vi "O2 RT Test.vi"() -> ()   [LabVIEW 2011]
uses:
  <vilib>/Platform/TimedLoop/XDataNode/timing_clust.ctl
  <vilib>/Platform/TimedLoop/XDataNode/nitl_modes.ctl
  <vilib>/Platform/TimedLoop/XDataNode/wakeup.ctl
  <vilib>/FPGAPlugInAG/cRIO-9074/niLvFpga_Open_cRIO-9074.vi
  <vilib>/rvi/interface/common/dynamic/niFpgaDynamicAddResources.vi
  <vilib>/Utility/error.llb/Error Cluster From Error Code.vi
  <vilib>/rvi/errors/niLvFpgaAdjustHostInterfaceError.vi
  <vilib>/FPGAPlugInAG/Dynamic/niLvFpga_Close_Dynamic.vi
  <vilib>/Platform/TimedLoop/XDataNode/XDataNode.xnode
  <vilib>/rvi/interface/nirviOpenFPGA/nirviOpenFPGA.xnode
  FPGA Bitfiles/MAXCAT_FPGATarget2_O2test_344E535A.lvbitx
  O2 test.vi
  <vilib>/rvi/interface/nirviReadWriteControl/nirviReadWriteControl.xnode
  <vilib>/rvi/interface/nirviCloseFPGA/nirviCloseFPGA.xnode
  <vilib>/Platform/TimedLoop/XDataNode/XDNodeRunTimeDep.lvlib
  NiFpgaLv.dll
  <vilib>/rvi/interface/Simulation/niFpgaSimulationCallBeginRW.vi
panel:
  out "FPGA Error Out":errorcluster
  in  "Stop":bool
  out "Lambda Chart":T1(graph)
  in  "UEGOModuleEnable":bool
  in  "UEGO Back Pressure (bar)":T2={"UEGO1BackPressure (bar)"=1.013, "UEGO2BackPressure (bar)"=1.013}
  in  "SensorEnable":T3
  out "UEGO Sensor Results":T4={"UEGO1Lambda"=1.0036743, "UEGO1Phi"=1.0, "UEGO1AFRatio"=14.7, "UEGO1Ip (mA)"=0.0, "UEGO2Lambda"=1.0033587, "UEGO2Phi"=1.0, "UEGO2AFRatio"=14.7, "UEGO2Ip (mA)"=0.0} {"UEGO1Lambda" scale=0.7..1.3; "UEGO2Lambda" scale=0.7..1.3}
  out "EGO Sensor Results":T5 {"EGO4Status" items=["COLD SENSOR", "FOULED SENSOR", "RICH", "LEAN"]; "EGO3Status" items=["COLD SENSOR", "FOULED SENSOR", "RICH", "LEAN"]; "EGO2Status" items=["COLD SENSOR", "FOULED SENSOR", "RICH", "LEAN"]; "EGO1Status" items=["COLD SENSOR", "FOULED SENSOR", "RICH", "LEAN"]}
  out "UEGO Temperature (C)":T6
  out "UEGO Heater Duty Cycle (%)":T7
  out "UEGO Diagnostics":T8={"ModulePresent"=FALSE, "UEGO1SensorFault"=63, "UEGO2SensorFault"=63, "UEGO1HeaterFault"=192, "UEGO2HeaterFault"=192, "UEGOFuseStatus"=0, "Battery (V)"=0.0} {"UEGOFuseStatus" items=["FUSE OK", "FUSE BLOWN"]; "UEGO2SensorFault" items=["NO FAULT"=63, "SHORT TO GND OR BATT"=0]; "UEGO2HeaterFault" items=["SHORT TO GROUND"=0, "OPEN CIRCUIT"=64, "SHORT TO BATTERY"=128, "NO FAULT"=192]; "UEGO1SensorFault" items=["NO FAULT"=63, "SHORT TO GND OR BATT"=0]; "UEGO1HeaterFault" items=["SHORT TO GROUND"=0, "OPEN CIRCUIT"=64, "SHORT TO BATTERY"=128, "NO FAULT"=192]}
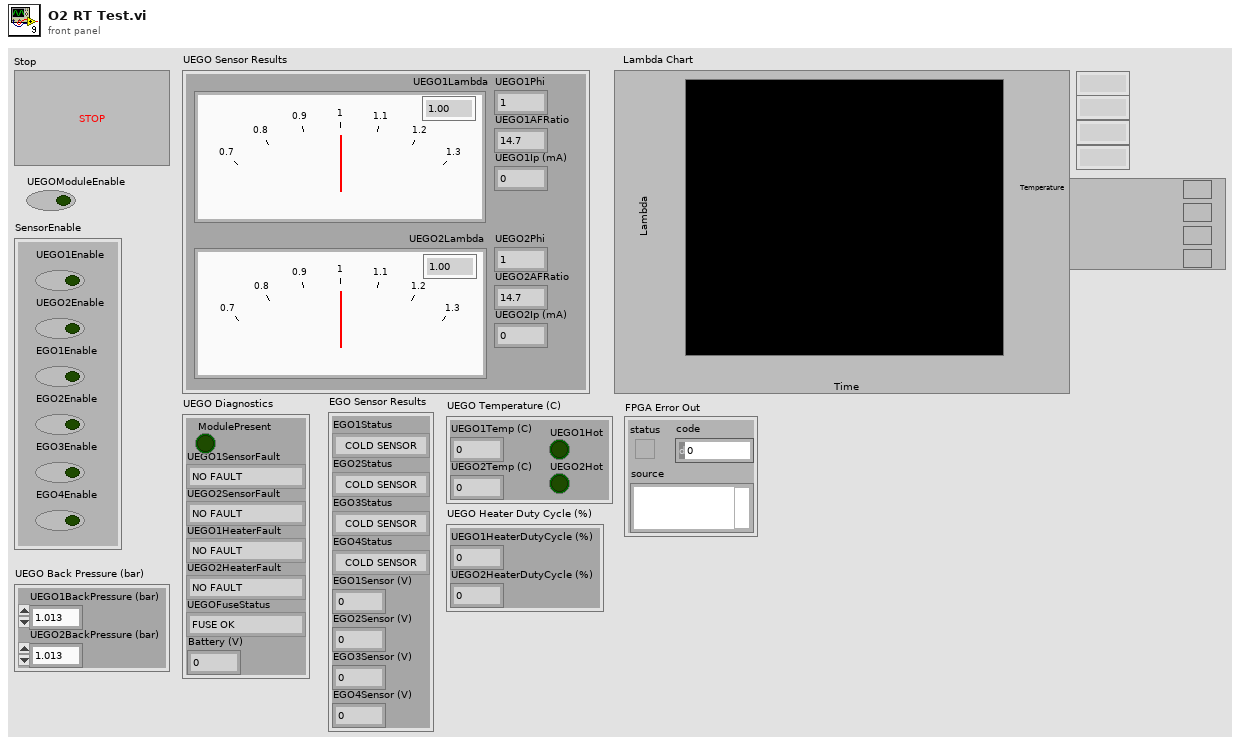
[diagram p1: front panel]
types:
  T1 = cluster{"UEGO1Lambda":sgl, "UEGO2Lambda":sgl, "UEGO1Temp (C)":sgl, "UEGO2Temp (C)":sgl}
  T2 = cluster{"UEGO1BackPressure (bar)":sgl, "UEGO2BackPressure (bar)":sgl}
  T3 = cluster{"UEGO1Enable":bool, "UEGO2Enable":bool, "EGO1Enable":bool, "EGO2Enable":bool, "EGO3Enable":bool, "EGO4Enable":bool}
  T4 = cluster{"UEGO1Lambda":sgl, "UEGO1Phi":sgl, "UEGO1AFRatio":sgl, "UEGO1Ip (mA)":sgl, "UEGO2Lambda":sgl, "UEGO2Phi":sgl, "UEGO2AFRatio":sgl, "UEGO2Ip (mA)":sgl}
  T5 = cluster{"EGO1Status":u8, "EGO2Status":u8, "EGO3Status":u8, "EGO4Status":u8, "EGO1Sensor (V)":sgl, "EGO2Sensor (V)":sgl, "EGO3Sensor (V)":sgl, "EGO4Sensor (V)":sgl}
  T6 = cluster{"UEGO1Temp (C)":sgl, "UEGO2Temp (C)":sgl, "UEGO1Hot":bool, "UEGO2Hot":bool}
  T7 = cluster{"UEGO1HeaterDutyCycle (%)":sgl, "UEGO2HeaterDutyCycle (%)":sgl}
  T8 = cluster{"ModulePresent":bool, "UEGO1SensorFault":u8, "UEGO2SensorFault":u8, "UEGO1HeaterFault":u8, "UEGO2HeaterFault":u8, "UEGOFuseStatus":u8, "Battery (V)":sgl}
  T9 = typedef "XDNodeRunTimeDep.lvlib/timing_clust.ctl" = cluster{"Expected End [f-1]":u64, "Actual End [f-1]":u64, "Finished Late? [f-1]":bool, "Expected End [i-1]":u64, "Actual End [i-1]":u64, "Finished Late? [i-1]":bool, "Expected Start [i]":u64, "Actual Start [i]":u64, "Expected Start [f]":u64, "Actual Start [f]":u64, "Source Name":string, "Structure Name":string, "Period":i64, "Deadline":i64, "Offset":i64, "Start":i64, "Priority":i32, "Timeout":i32, "Mode":T10, "Wakeup Reason":T11, "Error":errorcluster, "Source Type":string, "Secondary Source Type":string, "Global End Time":u64, "Global Start Time":u64, "Frame Duration":u64, "Iteration Duration":u64, "Assigned CPU":i32, "I/O Scan Engine Mode":u32}
  T10 = typedef "XDNodeRunTimeDep.lvlib/nitl_modes.ctl" = enum32{"No Change", "Process missed periods, maintain original phase", "Discard missed periods, maintain original phase", "Process missed periods, ignore original phase", "Discard missed periods, ignore original phase"}
  T11 = typedef "XDNodeRunTimeDep.lvlib/wakeup.ctl" = enum32{"Normal", "Aborted", "Asynchronous wakeup", "Timing source error", "Timed loop error", "Timeout"}
  T12 = cluster{"Stoich A/F Ratio":sgl, "IpArray (mA)":sgl[], "LambdaArray":sgl[]}
  T13 = cluster{"UEGO1Diag":u8, "UEGO2Diag":u8, "UEGO1Sensor":i16, "UEGO2Sensor":i16, "UEGO1Heater":i16, "UEGO2Heater":i16, "UEGO1AmpOffset":i16, "UEGO2AmpOffset":i16, "UEGO1RIOffset":i16, "UEGO2RIOffset":i16, "UEGO1HeaterGain":i16, "UEGO2HeaterGain":i16, "Fuse":i16, "EGO1Sensor":i16, "EGO2Sensor":i16, "EGO3Sensor":i16, "EGO4Sensor":i16, "Battery":i16, "ModulePresent":bool, "UEGO1ID":u8, "UEGO2ID":u8}
  T14 = cluster{"ModuleEnable":bool, "WatchdogIn":bool, "UEGO1Hot":bool, "UEGO2Hot":bool, "Cal1Request":bool, "Cal2Request":bool, "UEGOHeaterPeriod":u16, "UEGO1HeaterPulseWidth":u16, "UEGO2HeaterPulseWidth":u16}
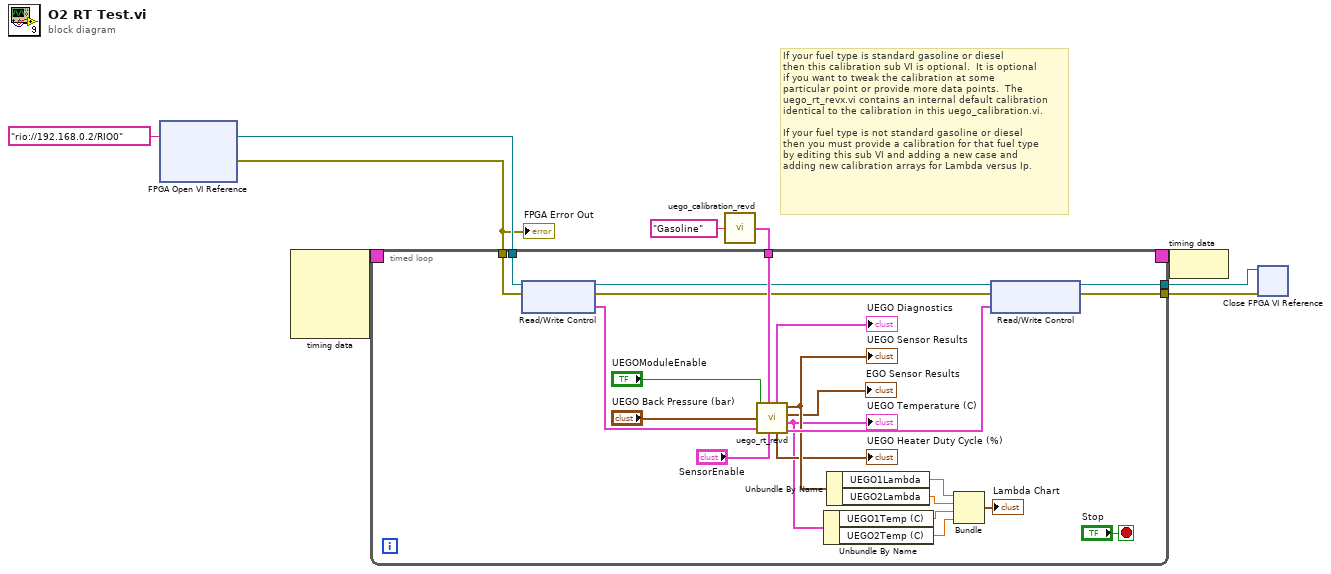
[diagram p0: block diagram]
diagram:
  # "If your fuel type is standard gasoline or diesel\nthen this calibration sub VI is optional.  It is optional \nif you want to tweak the calibration at some \nparticular point or provide more data points.  The \nuego_rt_revx.vi contains an internal default calibration\nidentical to the calibration in this uego_calibration.vi.\n\nIf your fuel type is not standard gasoline or diesel\nthen you must provide a calibration for that fuel type\nby editing this sub VI and adding a new case and \nadding new calibration arrays for Lambda versus Ip."
  n1 = xnode "FPGA Open VI Reference"("resource name"=tag "rio://192.168.0.2/RIO0") -> ("FPGA VI Reference Out"=w6:refnum<k20>, "error out"=w5:errorcluster)  [unwired: 1 in]
  "FPGA Error Out" <- w5
  n2 = node-c288() -> (w9:T9)  [unwired: 4 out]
  n3 = call <vilib>:"uego_calibration_revd.vi"("Fuel Selection"="Gasoline") -> ("UEGOCalibration"=w7:T12)
  n4 = timed-loop {
    tunnel: w5 -> [w29]
    tunnel: w7 -> [w31]
    tunnel: w6 -> [w32]
    timing-out: [_] -> w8
    timing: w9 -> [_]
    tunnel: [w20] -> w4
    tunnel: [w19] -> w3
    stop <- "Stop" stop-if-true
    n5 = xnode "Read/Write Control"("FPGA VI Reference In"=w32, "error in"=w29) -> ("FPGA VI Reference Out"=w30:refnum<k20>, "error out"=w28:errorcluster, "UEGOData"=w22:T13)
    n6 = call <vilib>:"uego_rt_revd.vi"("UEGOModuleEnable"="UEGOModuleEnable", "UEGOCalibration"=w31, "UEGO Back Pressure (bar)"="UEGO Back Pressure (bar)", "UEGOData (From FPGA)"=w22, "SensorEnable"="SensorEnable") -> ("UEGO Diagnostics"=→"UEGO Diagnostics":T8, "UEGO Sensor Results"=w21:T4, "EGO Sensor Results"=→"EGO Sensor Results":T5, "UEGO Heater Duty Cycle (%)"=→"UEGO Heater Duty Cycle (%)":T7, "UEGO Temperature (C)"=w13:T6, "UEGOControl (To FPGA)"=w23:T14)
    "UEGO Sensor Results" <- w21
    "UEGO Temperature (C)" <- w13
    n7 = Unbundle By Name(w13) -> ("UEGO1Temp (C)"=w12:sgl, "UEGO2Temp (C)"=w11:sgl)
    n8 = Unbundle By Name(w21) -> ("UEGO1Lambda"=w25:sgl, "UEGO2Lambda"=w24:sgl)
    n9 = Bundle("UEGO1Lambda"=w25, "UEGO2Lambda"=w24, "UEGO1Temp (C)"=w12, "UEGO2Temp (C)"=w11) -> (→"Lambda Chart":T1)  [unwired: 1 out]
    n10 = xnode "Read/Write Control"("FPGA VI Reference In"=w30, "error in"=w28, "UEGOControl"=w23) -> ("FPGA VI Reference Out"=w19:refnum<k20>, "error out"=w20:errorcluster)
  }
  n11 = node-c288(w8) -> ()
  n12 = xnode "Close FPGA VI Reference"("FPGA VI Reference In"=w3, "error in"=w4) -> ()  [unwired: 1 out]
